vi "QuickProfile_V3.vi"(7 "Image IN":sgl[][](array[numeric]), 11 "Pixel Size (nm)":dbl) -> ()   [LabVIEW 2014]
uses:
  <vilib>/Utility/file.llb/Write To Spreadsheet File (DBL).vi
panel:
  in  "ROI Size (Pixles)":dbl(slide)=1.0 min=1.0 max=500.0 step=1.0 scale=0.0..100.0 scale format="%#_3g"
  in  "Open Image":bool
  in  "Save ROI":bool
  out "Lorentzian Fit Width (nm)":dbl
  out "Gaussian Fit Width Y (nm)":dbl
  out "Gaussian Fit Width X (nm)":dbl
  out "Constant Y Slice":cluster{"X Values":dbl[], sgl[]}[](graph)
  out "Constant X Slice":cluster{"X Values":dbl[], sgl[]}[](graph)
  in  "Fit ROI":bool
  out "Gaussian Fit":dbl[][](graph)
  out "Lorentzian Fit":dbl[][](graph)
  out "Current ROI":sgl[][](graph)
  in  "Quit":bool
  out "Image Display":sgl[][](graph)
  # "Constant Y"
  # "Constant X"
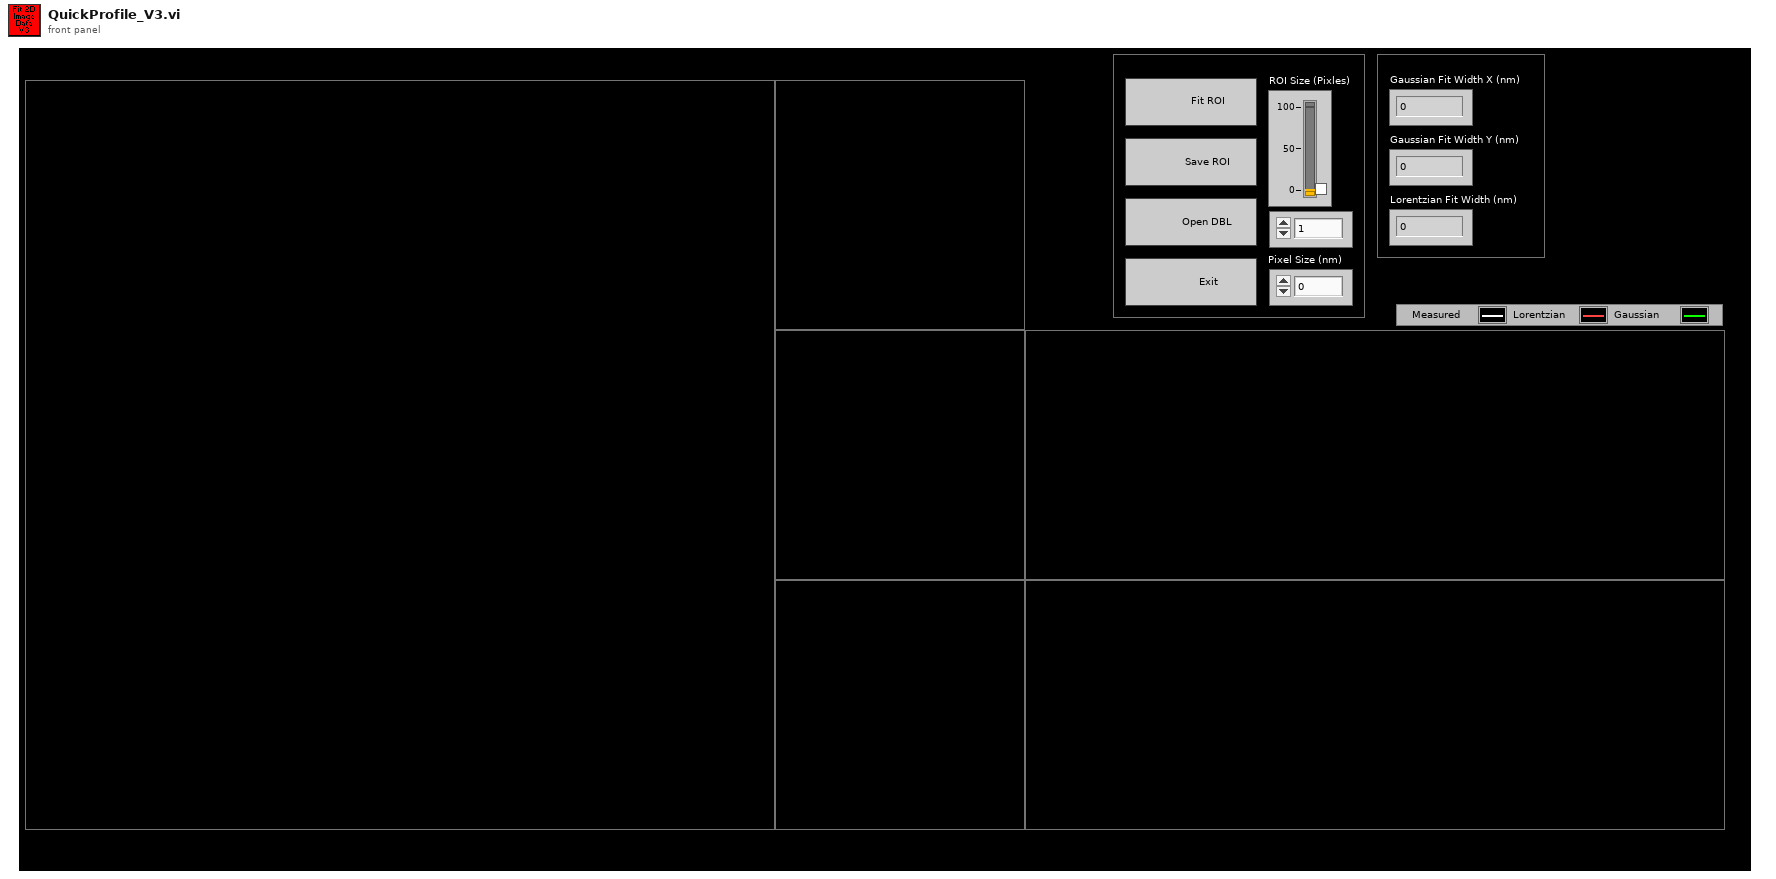
[diagram p1: front panel]
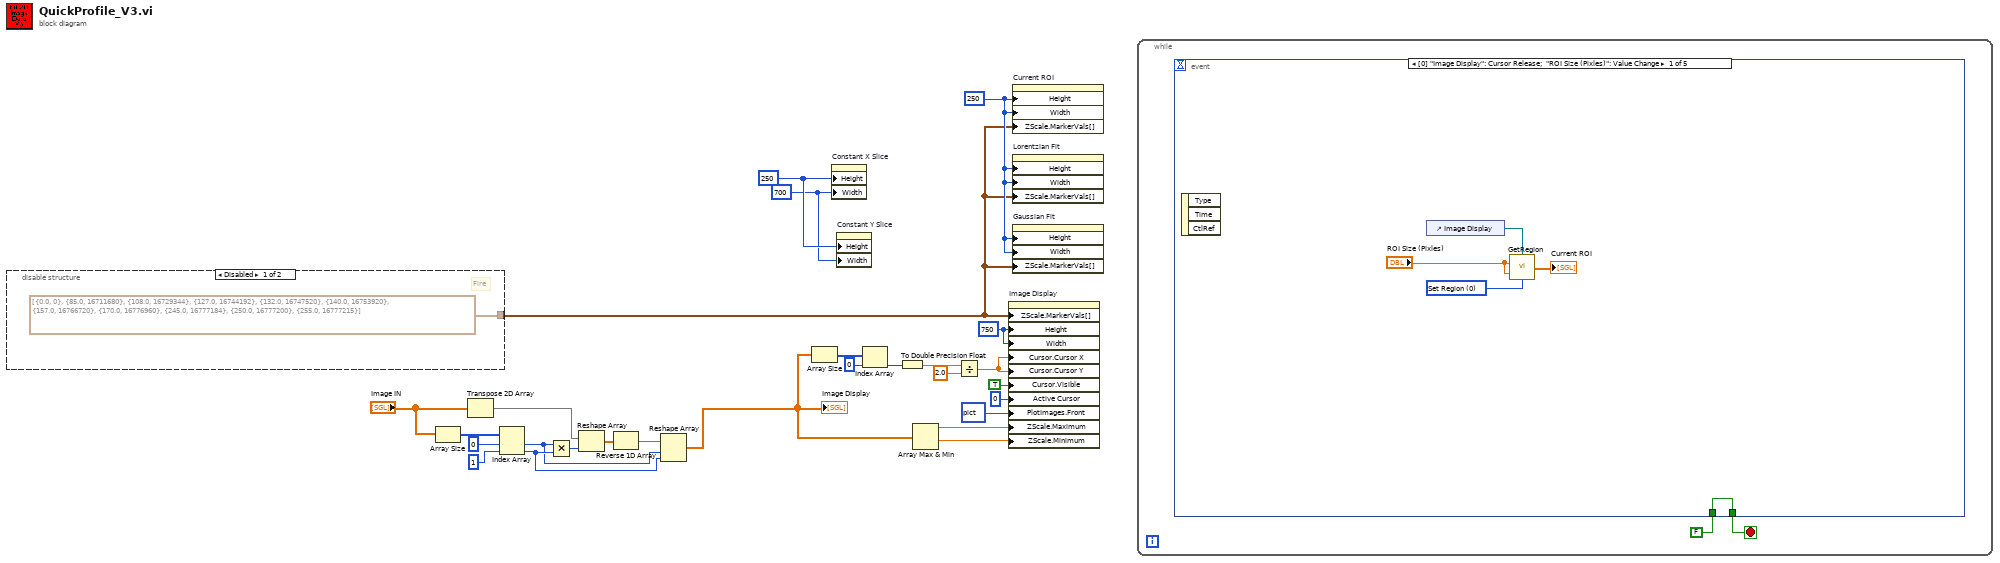
[diagram p0: block diagram]
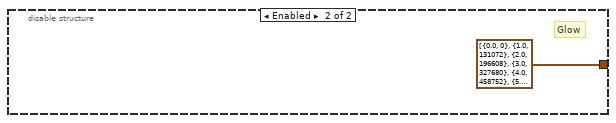
[diagram p2: hidden frame]
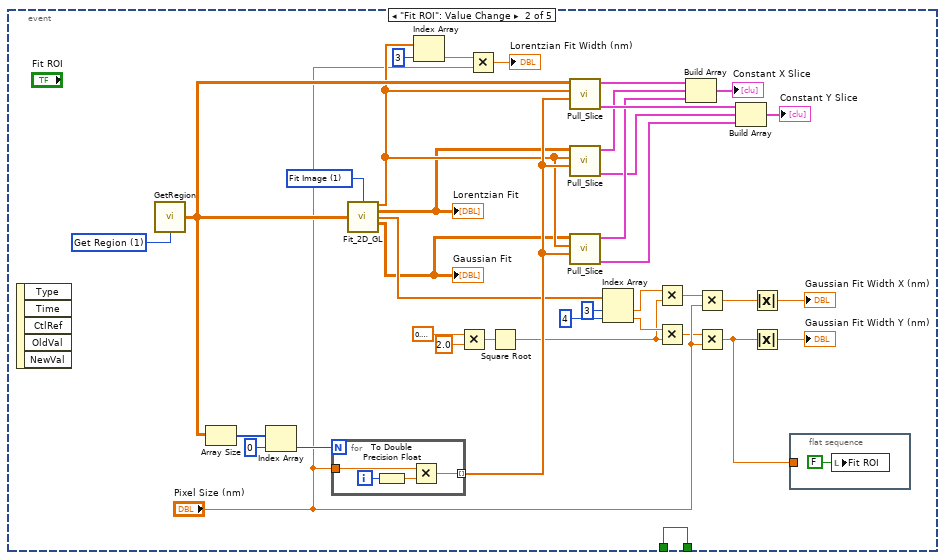
[diagram p3: hidden frame]
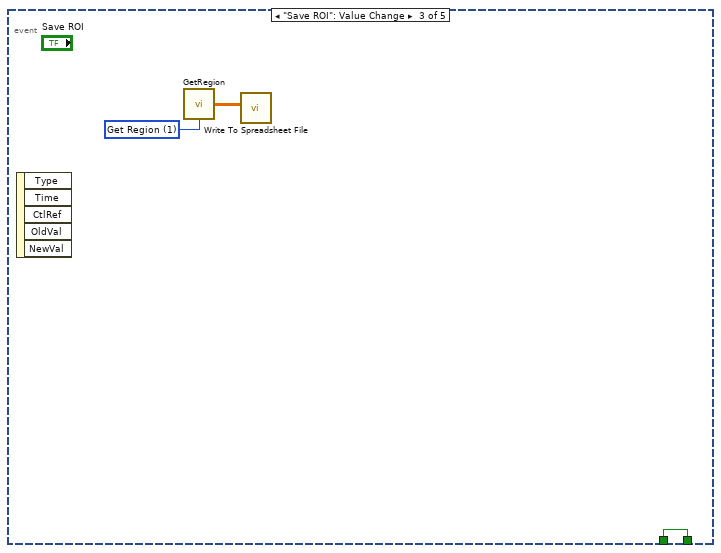
[diagram p4: hidden frame]
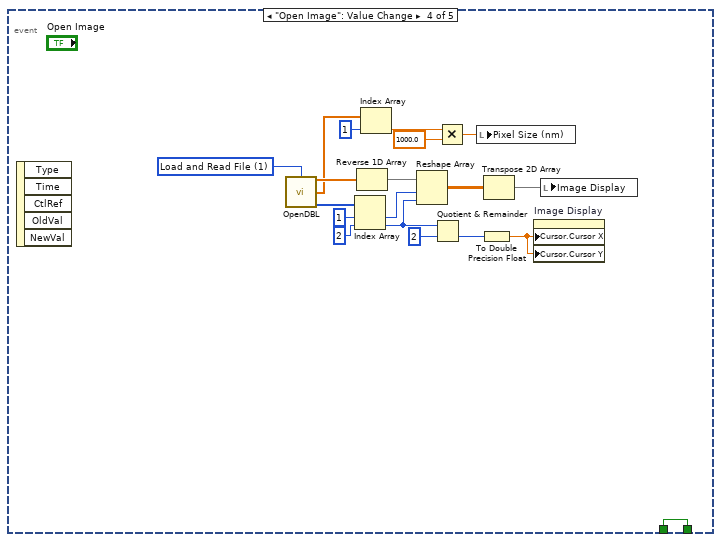
[diagram p5: hidden frame]
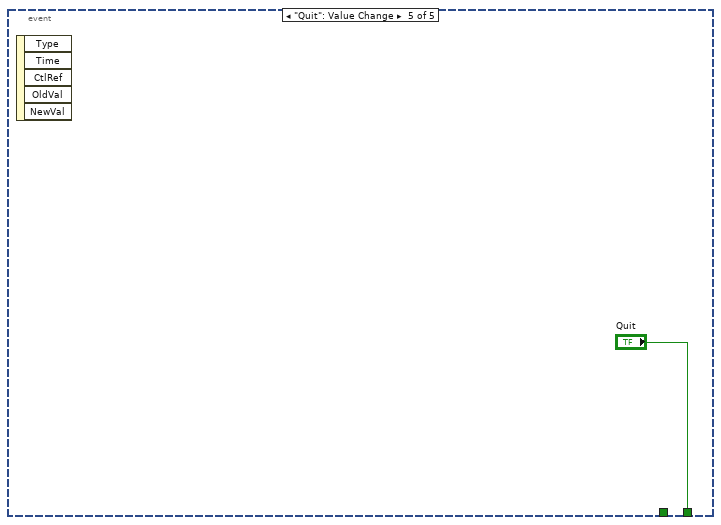
[diagram p6: hidden frame]
diagram:
  w20 = u32 700 ("Plot Area:Size:Width")
  w21 = u32 250 ("Plot Area:Size:Height")
  w23 = u32 250 ("Plot Area:Size:Height")
  w27 = u32 750 ("Plot Area:Size:Height")
  n1 = disable-structure shown="Disabled" {
    disable-tunnel: [cluster{dbl, u32}[] [{0.0, 0}, {85.0, 16711680}, {108.0, 16729344}, {127.0, 16744192}, {132.0, 16747520}, {140.0, 16753920}, {157.0, 16766720}, {170.0, 16776960}, {245.0, 16777184}, {250.0, 16777200}, {255.0, 16777215}] ("Z Scale.Marker Values[]") cluster{dbl, u32}[] [{0.0, 0}, {1.0, 131072}, {2.0, 196608}, {3.0, 327680}, {4.0, 458752}, {5.0, 589824}, {6.0, 720896}, {7.0, 851971}, {8.0, 983043}, {9.0, 1114115}, {10.0, 1245187}, {11.0, 1376259}, {12.0, 1507331}, {13.0, 1638403}, {14.0, 1769475}, {15.0, 1769479}, {16.0, 2031623}, {17.0, 2162695}, {18.0, 2293767}, {19.0, 2424839}, {20.0, 2555911}, {21.0, 2686983}, {22.0, 2818055}, {23.0, 2949127}, {24.0, 3080203}, {25.0, 3211275}, {26.0, 3342347}, {27.0, 3473419}, {28.0, 3604491}, {29.0, 3735563}, {30.0, 3866635}, {31.0, 3867403}, {32.0, 4129547}, {33.0, 4260619}, {34.0, 4391691}, {35.0, 4522763}, {36.0, 4653839}, {37.0, 4784911}, {38.0, 4915983}, {39.0, 5178127}, {40.0, 5309199}, {41.0, 5440271}, {42.0, 5571343}, {43.0, 5702415}, {44.0, 5703439}, {45.0, 5965583}, {46.0, 6096655}, {47.0, 6227727}, {48.0, 6358799}, {49.0, 6489871}, {50.0, 6620943}, {51.0, 6752015}, {52.0, 6883087}, {53.0, 7015183}, {54.0, 7146255}, {55.0, 7277327}, {56.0, 7408399}, {57.0, 7539471}, {58.0, 7670543}, {59.0, 7801615}, {60.0, 8063759}, {61.0, 8194831}, {62.0, 8326927}, {63.0, 8457999}, {64.0, 8589075}, {65.0, 8720147}, {66.0, 8851219}, {67.0, 8982291}, {68.0, 9113363}, {69.0, 9114387}, {70.0, 9376531}, {71.0, 9507603}, {72.0, 9638675}, {73.0, 9769747}, {74.0, 9901843}, {75.0, 10032915}, {76.0, 10163987}, {77.0, 10229523}, {78.0, 10295059}, {79.0, 10427155}, {80.0, 10558227}, {81.0, 10689299}, {82.0, 10820371}, {83.0, 10886931}, {84.0, 10952467}, {85.0, 11083539}, {86.0, 11214611}, {87.0, 11215635}, {88.0, 11477779}, {89.0, 11543315}, {90.0, 11608851}, {91.0, 11740947}, {92.0, 11806483}, {93.0, 11872019}, {94.0, 12004115}, {95.0, 12135187}, {96.0, 12266259}, {97.0, 12267283}, {98.0, 12398355}, {99.0, 12529427}, {100.0, 12530451}, {101.0, 12595987}, {102.0, 12530451}, {103.0, 12793619}, {104.0, 12794131}, {105.0, 12794643}, {106.0, 13056787}, {107.0, 13057299}, {108.0, 13057811}, {109.0, 13188883}, {110.0, 13320979}, {111.0, 13386515}, {112.0, 13452563}, {113.0, 13584147}, {114.0, 13584659}, {115.0, 13585171}, {116.0, 13585683}, {117.0, 13717267}, {118.0, 13848339}, {119.0, 13849363}, {120.0, 13849875}, {121.0, 13850387}, {122.0, 13981459}, {123.0, 14113555}, {124.0, 14114067}, {125.0, 14114579}, {126.0, 14115091}, {127.0, 14246675}, {128.0, 14377747}, {129.0, 14378771}, {130.0, 14379283}, {131.0, 14379539}, {132.0, 14379795}, {133.0, 14380819}, {134.0, 14511891}, {135.0, 14643987}, {136.0, 14644503}, {137.0, 14645015}, {138.0, 14645527}, {139.0, 14646039}, {140.0, 14646551}, {141.0, 14778135}, {142.0, 14909207}, {143.0, 14910231}, {144.0, 14910747}, {145.0, 14911259}, {146.0, 14911771}, {147.0, 14912283}, {148.0, 14912797}, {149.0, 15044383}, {150.0, 15175455}, {151.0, 15175967}, {152.0, 15176479}, {153.0, 15176991}, {154.0, 15177507}, {155.0, 15178019}, {156.0, 15178531}, {157.0, 15310115}, {158.0, 15441701}, {159.0, 15441959}, {160.0, 15442215}, {161.0, 15442727}, {162.0, 15443243}, {163.0, 15443755}, {164.0, 15444269}, {165.0, 15444783}, {166.0, 15444783}, {167.0, 15576367}, {168.0, 15707953}, {169.0, 15708467}, {170.0, 15708979}, {171.0, 15708981}, {172.0, 15708983}, {173.0, 15710011}, {174.0, 15710523}, {175.0, 15711037}, {176.0, 15711039}, {177.0, 15711553}, {178.0, 15843139}, {179.0, 15974213}, {180.0, 15974215}, {181.0, 15974217}, {182.0, 15974219}, {183.0, 15975755}, {184.0, 15976271}, {185.0, 15976785}, {186.0, 15977299}, {187.0, 15977301}, {188.0, 15977815}, {189.0, 15978327}, {190.0, 15978331}, {191.0, 16109917}, {192.0, 16241503}, {193.0, 16241505}, {194.0, 16242019}, {195.0, 16242535}, {196.0, 16242537}, {197.0, 16242539}, {198.0, 16243563}, {199.0, 16243567}, {200.0, 16244081}, {201.0, 16244595}, {202.0, 16244599}, {203.0, 16244601}, {204.0, 16244603}, {205.0, 16245627}, {206.0, 16245631}, {207.0, 16245633}, {208.0, 16246147}, {209.0, 16246663}, {210.0, 16377735}, {211.0, 16508811}, {212.0, 16508815}, {213.0, 16509839}, {214.0, 16509843}, {215.0, 16509845}, {216.0, 16509847}, {217.0, 16510361}, {218.0, 16510875}, {219.0, 16510879}, {220.0, 16510881}, {221.0, 16510883}, {222.0, 16511399}, {223.0, 16511911}, {224.0, 16511915}, {225.0, 16511917}, {226.0, 16511919}, {227.0, 16511923}, {228.0, 16512437}, {229.0, 16512951}, {230.0, 16512955}, {231.0, 16512957}, {232.0, 16512959}, {233.0, 16512961}, {234.0, 16512963}, {235.0, 16512967}, {236.0, 16513481}, {237.0, 16513995}, {238.0, 16513999}, {239.0, 16514001}, {240.0, 16514003}, {241.0, 16514005}, {242.0, 16514007}, {243.0, 16514011}, {244.0, 16514013}, {245.0, 16514015}, {246.0, 16514019}, {247.0, 16514021}, {248.0, 16514023}, {249.0, 16514027}, {250.0, 16514029}, {251.0, 16514031}, {252.0, 16514035}, {253.0, 16514037}, {254.0, 16514039}, {255.0, 16514043}] ("Z Scale.Marker Values[]")] -> w22
    frame Disabled {
      # "Fire"
    }
    frame Enabled {
      # "Glow"
    }
  }
  n2 = Array Size(array="Image IN") -> (size(s)=w11:i32[])
  n3 = Transpose 2D Array(2D array="Image IN") -> (transposed array=w2:sgl[][])
  n4 = Index Array(array=w11, index #1=0 ("index"), index #2=1 ("index")) -> (element #1=w3:i32, element #2=w4:i32)
  n5 = Multiply(x=w3, y=w4) -> (x*y=w9:i32)
  n6 = Reshape Array(w2, w9) -> (w6:sgl[])
  n7 = Reverse 1D Array(array=w6) -> (reversed array=w5:sgl[])
  n8 = Reshape Array(w5, w3, w4) -> (w1:sgl[][])
  "Image Display" <- w1
  n9 = Array Size(array=w1) -> (size(s)=w17:i32[])
  n10 = property on="Constant X Slice" class="XYGraph (strict)"("Height"=w21, "Width"=w20) -> ()  [unwired: 2 in, 2 out]
  n11 = property on="Constant Y Slice" class="XYGraph (strict)"("Height"=w21, "Width"=w20) -> ()  [unwired: 2 in, 2 out]
  n12 = Index Array(array=w17, index=0) -> (element=w15:i32)
  n13 = To Double Precision Float(number=w15) -> (double precision float=w13:dbl)
  n14 = Array Max & Min(array=w1) -> (max value=w19:sgl, min value=w18:sgl)  [unwired: 2 out]
  n15 = Divide(x=w13, y=2.0) -> (x/y=w12:dbl)
  n16 = property on="Image Display" class="IntGraph (strict)"("ZScale.MarkerVals[]"=w22, "Height"=w27, "Width"=w27, "Cursor.Cursor X"=w12, "Cursor.Cursor Y"=w12, "Cursor.Visible"=TRUE, "Active Cursor"=u32 0, "PlotImages.Front"=picture data[5B] ("Plot Images:Front"), "ZScale.Maximum"=w19, "ZScale.Minimum"=w18) -> ()  [unwired: 2 in, 2 out]
  n17 = property on="Current ROI" class="IntGraph (strict)"("Height"=w23, "Width"=w23, "ZScale.MarkerVals[]"=w22) -> ()  [unwired: 2 in, 2 out]
  n18 = property on="Lorentzian Fit" class="IntGraph (strict)"("Height"=w23, "Width"=w23, "ZScale.MarkerVals[]"=w22) -> ()  [unwired: 2 in, 2 out]
  n19 = property on="Gaussian Fit" class="IntGraph (strict)"("Height"=w23, "Width"=w23, "ZScale.MarkerVals[]"=w22) -> ()  [unwired: 2 in, 2 out]
  n20 = while {
    stop <- w31 stop-if-true
    n21 = event shown="[0] \"Image Display\": Cursor Release;  \"ROI Size (Pixles)\": Value Change" {
      selector: _ -> [_ _ _ _ _]
      dyn-events: _ -> [_ _ _ _ _]
      timeout: _ -> [_ _ _ _ _]
      tunnel: [w35 w74 w81 w101 "Quit"] -> w31
      tunnel: FALSE -> [w35 w74 w81 w101 _]
      event "Image Display": Cursor Release; "ROI Size (Pixles)": Value Change {
        w34 = u16 0 items=["Set Region", "Get Region"] ("Action")
        n22 = event-data() -> ()  [unwired: 1 in, 3 out]
        n23 = control-ref of="Image Display"() -> (w36:refnum<vi>)
        n24 = call "GetRegion.vi"("IntGraph REF"=w36, "Y Width (PX)"="ROI Size (Pixles)", "X Width (PX)"="ROI Size (Pixles)", "Action"=w34) -> ("Region Out"=→"Current ROI":sgl[][])  [unwired: 11 in]
      }
      event "Fit ROI": Value Change {
        w72 = u16 1 items=["Read Fit Data", "Fit Image"] ("Action")
        w73 = u16 1 items=["Set Region", "Get Region"] ("Action")
        n25 = event-data() -> ()  [unwired: 1 in, 5 out]
        n26 = call "GetRegion.vi"("Action"=w73) -> ("Region Out"=w62:sgl[][])  [unwired: 14 in]
        n27 = Array Size(array=w62) -> (size(s)=w71:i32[])
        n28 = Index Array(array=w71, index=0) -> (element=w69:i32)
        n29 = for {
          N: w69 -> [_]
          tunnel: "Pixel Size (nm)" -> [w78]
          tunnel: [w76] -> w68 mode=indexing
          i -> [w79]
          n30 = To Double Precision Float(number=w79) -> (double precision float=w77:dbl)
          n31 = Multiply(x=w78, y=w77) -> (x*y=w76:dbl)
        }
        n32 = call "Fit_2D_GL.vi"("Action"=w72, "Image IN"=w62) -> ("Lorentz Fit Parameters"=w57:dbl[], "Lorentzian Image"=w48:dbl[][], "Gaussian Fit Parameters"=w59:dbl[], "Gaussian Image"=w47:dbl[][])  [unwired: 9 in, 1 out]
        "Gaussian Fit" <- w47
        "Lorentzian Fit" <- w48
        n33 = Index Array(array=w57, index=3) -> (element=w53:dbl)
        n34 = Multiply(x=0.6931471805599453, y=2.0) -> (x*y=w42:dbl)
        n35 = Multiply(x=w53, y="Pixel Size (nm)") -> (x*y=→"Lorentzian Fit Width (nm)":dbl)
        n36 = Square Root(x=w42) -> (sqrt(x)=w39:dbl)
        n37 = call "Pull_Slice.vi"("X Values"=w68, "Fit Parameters"=w57, "ROI Image"=w62) -> ("Constant X Slice"=w67:cluster{"X Values":dbl[], sgl[]}, "Constant Y Slice"=w54:cluster{"X Values":dbl[], sgl[]})  [unwired: 7 in]
        n38 = call "Pull_Slice.vi"("X Values"=w68, "Fit Parameters"=w57, "ROI Image"=w48) -> ("Constant X Slice"=w64:cluster{"X Values":dbl[], sgl[]}, "Constant Y Slice"=w66:cluster{"X Values":dbl[], sgl[]})  [unwired: 7 in]
        n39 = call "Pull_Slice.vi"("X Values"=w68, "Fit Parameters"=w57, "ROI Image"=w47) -> ("Constant X Slice"=w63:cluster{"X Values":dbl[], sgl[]}, "Constant Y Slice"=w65:cluster{"X Values":dbl[], sgl[]})  [unwired: 7 in]
        n40 = Index Array(array=w59, index #1=3 ("index"), index #2=4 ("index")) -> (element #1=w46:dbl, element #2=w44:dbl)
        n41 = Multiply(x=w46, y=w39) -> (x*y=w45:dbl)
        n42 = Multiply(x=w44, y=w39) -> (x*y=w43:dbl)
        n43 = Build Array(w54, w66, w65) -> (→"Constant X Slice":cluster{"X Values":dbl[], sgl[]}[])
        n44 = Multiply(x=w45, y="Pixel Size (nm)") -> (x*y=w51:dbl)
        n45 = Multiply(x=w43, y="Pixel Size (nm)") -> (x*y=w49:dbl)
        n46 = Build Array(w67, w64, w63) -> (→"Constant Y Slice":cluster{"X Values":dbl[], sgl[]}[])
        n47 = Absolute Value(x=w51) -> (abs(x)=→"Gaussian Fit Width X (nm)":dbl)
        n48 = Absolute Value(x=w49) -> (abs(x)=→"Gaussian Fit Width Y (nm)":dbl)
        n49 = flat-sequence {
          tunnel: w49 -> [_]
          frame #0 {
            n50 = local write "Fit ROI"(FALSE ("Fit ROI")) -> ()
          }
        }
      }
      event "Save ROI": Value Change {
        w82 = u16 1 items=["Set Region", "Get Region"] ("Action")
        n51 = event-data() -> ()  [unwired: 1 in, 5 out]
        n52 = call "GetRegion.vi"("Action"=w82) -> ("Region Out"=w80:sgl[][])  [unwired: 14 in]
        n53 = call-poly <vilib>:"Write To Spreadsheet File.vi"("2D data"=w80) -> ()  [unwired: 7 in, 1 out]
      }
      event "Open Image": Value Change {
        w100 = u16 1 items=["Get Image", "Load and Read File"] ("Action")
        n54 = event-data() -> ()  [unwired: 1 in, 5 out]
        n55 = call "OpenDBL.vi"("Action"=w100) -> ("Image"=w99:sgl[], "Physical Length (Z, Y, X, t)"=w93:sgl[], "Dimensions (Z, Y, X, t)"=w98:i32[])  [unwired: 11 in, 1 out]
        n56 = Index Array(array=w98, index #1=1 ("index"), index #2=2 ("index")) -> (element #1=w95:i32, element #2=w88:i32)
        n57 = Reverse 1D Array(array=w99) -> (reversed array=w83:sgl[])
        n58 = Index Array(array=w93, index=1) -> (element=w91:sgl)
        n59 = Reshape Array(w83, w95, w88) -> (w94:sgl[][])
        n60 = Quotient & Remainder(x=w88, y=2) -> (floor(x/y)=w86:i32)  [unwired: 1 out]
        n61 = Multiply(x=w91, y=sgl 1000.0) -> (x*y=w89:sgl)
        n62 = local write "Pixel Size (nm)"(w89) -> ()
        n63 = To Double Precision Float(number=w86) -> (double precision float=w85:dbl)
        n64 = Transpose 2D Array(2D array=w94) -> (transposed array=w84:sgl[][])
        n65 = property on="Image Display" class="IntGraph (strict)"("Cursor.Cursor X"=w85, "Cursor.Cursor Y"=w85) -> ()  [unwired: 2 in, 2 out]
        n66 = local write "Image Display"(w84) -> ()
      }
      event "Quit": Value Change {
        n67 = event-data() -> ()  [unwired: 1 in, 5 out]
      }
    }
  }
